vi "RetrieveDiagPacket.vi"(8 "error in (no error)":errorcluster, 11 "Controller In":refnum<k24>) -> (0 "error out":errorcluster, 2 "ControllerDiagPacket":T1, 3 "Controller Out":refnum<k24>)   [LabVIEW 2010]
uses:
  c:/aerotech/controller/5.xx.xxx/ensemble/pc/labview/2010/bin/Aerotech.Ensemble.dll
  bin/Aerotech.Ensemble.dll
  ControllerDiagPacket.ctl
  AxisDiagPacket.ctl
  c:/aerotech/controller/5.xx.xxx/ensemble/pc/labview/2010/bin/Aerotech.Ensemble.LabVIEW.dll
  bin/Aerotech.Ensemble.LabVIEW.dll
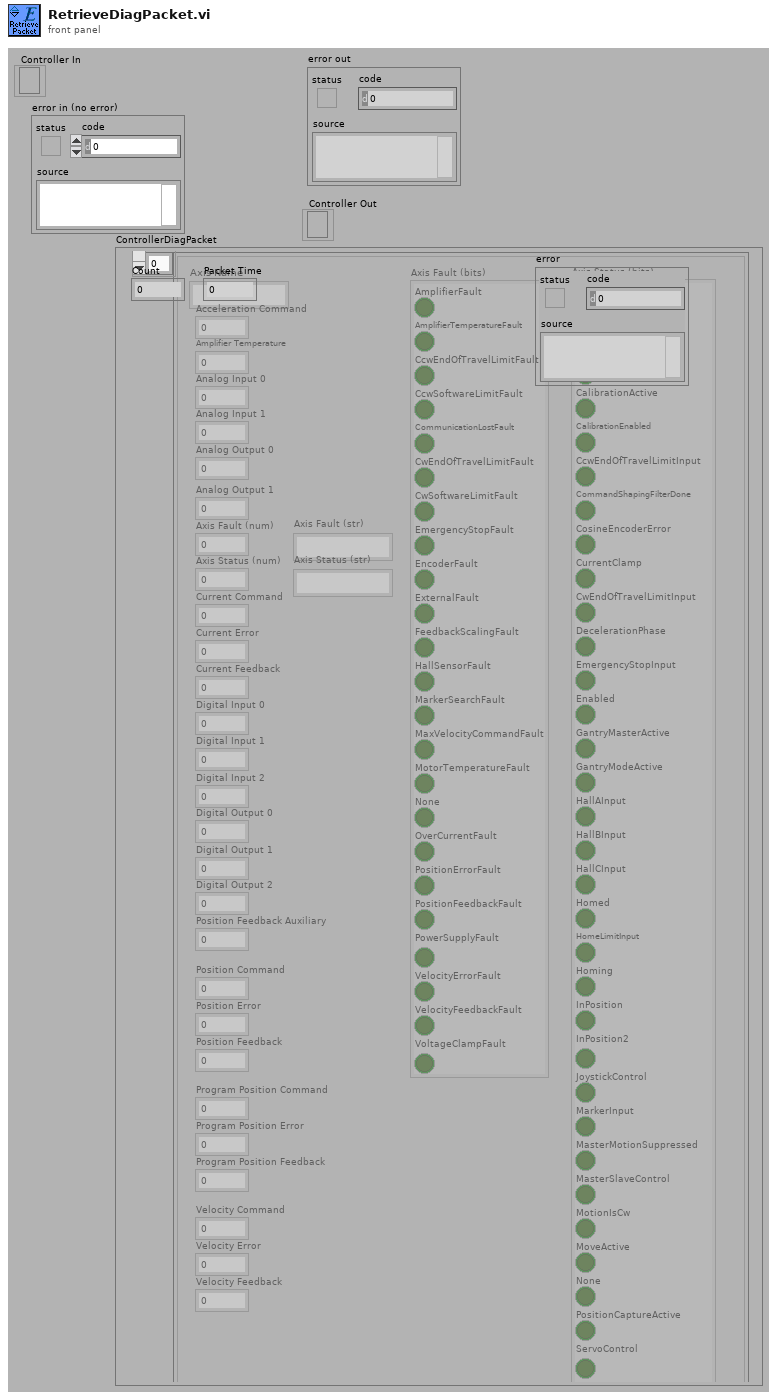
[diagram p1: front panel]
types:
  T1 = typedef "ControllerDiagPacket.ctl" = cluster{"Count":i32, "Packet Time":i64, "Axes":T2[], "error":errorcluster}
  T2 = typedef "AxisDiagPacket.ctl" = cluster{"Axis Name":string, "Acceleration Command":dbl, "Amplifier Temperature":sgl, "Analog Input 0":dbl, "Analog Input 1":dbl, "Analog Output 0":dbl, "Analog Output 1":dbl, "Axis Fault (num)":i32, "Axis Fault (str)":string, "Axis Fault (bits)":cluster{"AmplifierFault":bool, "AmplifierTemperatureFault":bool, "CcwEndOfTravelLimitFault":bool, "CcwSoftwareLimitFault":bool, "CommunicationLostFault":bool, "CwEndOfTravelLimitFault":bool, "CwSoftwareLimitFault":bool, "EmergencyStopFault":bool, "EncoderFault":bool, "ExternalFault":bool, "FeedbackScalingFault":bool, "HallSensorFault":bool, "MarkerSearchFault":bool, "MaxVelocityCommandFault":bool, "MotorTemperatureFault":bool, "None":bool, "OverCurrentFault":bool, "PositionErrorFault":bool, "PositionFeedbackFault":bool, "PowerSupplyFault":bool, "VelocityErrorFault":bool, "VelocityFeedbackFault":bool, "VoltageClampFault":bool}, "Axis Status (num)":i32, "Axis Status (str)":string, "Axis Status (bits)":cluster{"AccelerationPhase":bool, "AutofocusActive":bool, "BrakeOutput":bool, "CalibrationActive":bool, "CalibrationEnabled":bool, "CcwEndOfTravelLimitInput":bool, "CommandShapingFilterDone":bool, "CosineEncoderError":bool, "CurrentClamp":bool, "CwEndOfTravelLimitInput":bool, "DecelerationPhase":bool, "EmergencyStopInput":bool, "Enabled":bool, "GantryMasterActive":bool, "GantryModeActive":bool, "HallAInput":bool, "HallBInput":bool, "HallCInput":bool, "Homed":bool, "HomeLimitInput":bool, "Homing":bool, "InPosition":bool, "InPosition2":bool, "JoystickControl":bool, "MarkerInput":bool, "MasterMotionSuppressed":bool, "MasterSlaveControl":bool, "MotionIsCw":bool, "MoveActive":bool, "None":bool, "PositionCaptureActive":bool, "ServoControl":bool, "SineEncoderError":bool}, "Current Command":sgl, "Current Error":sgl, "Current Feedback":sgl, "Digital Input 0":i32, "Digital Input 1":i32, "Digital Input 2":i32, "Digital Output 0":i32, "Digital Output 1":i32, "Digital Output 2":i32, "Position Feedback Auxiliary":dbl, "Position Command":dbl, "Position Error":dbl, "Position Feedback":dbl, "Program Position Command":dbl, "Program Position Error":dbl, "Program Position Feedback":dbl, "Velocity Command":dbl, "Velocity Error":dbl, "Velocity Feedback":dbl}
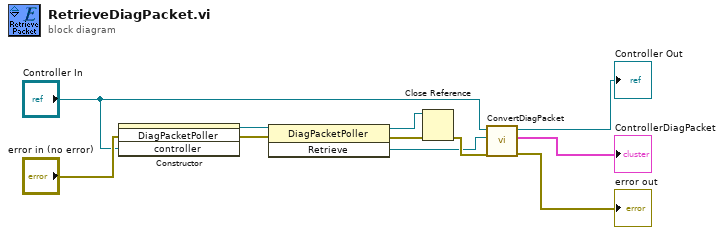
[diagram p0: block diagram]
diagram:
  n1 = constructor class="DiagPacketPoller"(error in="error in (no error)", "controller"="Controller In") -> (reference out=w9:refnum<k24>, error out=w10:errorcluster)  [unwired: 2 in, 2 out]
  n2 = invoke class="DiagPacketPoller" method="Retrieve"(reference=w9, error in=w10) -> (reference out=w5:refnum<k24>, error out=w7:errorcluster, "Retrieve"=w1:refnum<k24>)  [unwired: 1 in]
  n3 = Close Reference(reference=w5, error in (no error)=w7) -> (error out=w6:errorcluster)
  n4 = call "ConvertDiagPacket.vi"("error in (no error)"=w6, ".NET data in"=w1, "controller in"="Controller In") -> ("error out"=→"error out":errorcluster, "LabVIEW data out"=→"ControllerDiagPacket":T1, "controller out"=→"Controller Out":refnum<k24>)  [unwired: 6 in]
